vi "WinCI Query File Status.vi"(8 "error in (no error)":errorcluster, 10 "files":path[](array[path]), 11 "source control reference in":T2) -> (0 "error out":errorcluster, 1 "file status":T1[](array[typedef]), 2 "status message":string, 3 "source control reference out":T2)   [LabVIEW 2020, in "NI_SCC_WinCI.lvlib"]
uses:
  <vilib>/SourceControl/Providers/WinCI/NI_SCC_WinCI.lvlib
  <vilib>/SourceControl/sccapi/SCCAPI Refnum.ctl
  <vilib>/SourceControl/Providers/WinCI/WinCI SCC File Status.ctl
  <vilib>/SourceControl/support/SCCSup Message Strings GLBL.vi
  <vilib>/SourceControl/sccapi/NI_SCC.lvlib
panel:
  in  "null file status TD":T1
  out "raw file status":i32[](array[numeric])
  out "result":i32
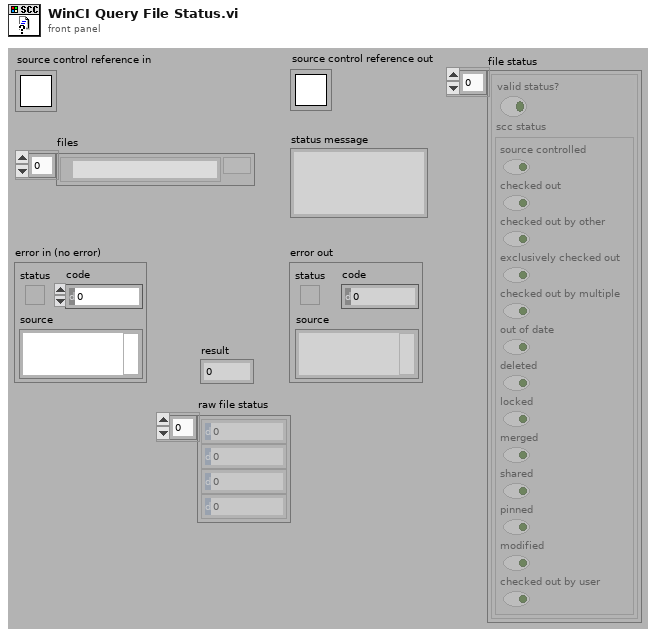
[diagram p1: front panel]
types:
  T1 = typedef "NI_SCC_WinCI.lvlib/WinCI SCC File Status.ctl" = cluster{"valid status?":bool, "scc status":cluster{"source controlled":bool, "checked out":bool, "checked out by other":bool, "exclusively checked out":bool, "checked out by multiple":bool, "out of date":bool, "deleted":bool, "locked":bool, "merged":bool, "shared":bool, "pinned":bool, "modified":bool, "checked out by user":bool}}
  T2 = typedef "NI_SCC.lvlib/SCCAPI Refnum.ctl" = refnum<k1>
  T3 = cluster{"Boolean array[0]":bool, "Boolean array[1]":bool, "Boolean array[2]":bool, "Boolean array[3]":bool, "Boolean array[4]":bool, "Boolean array[5]":bool, "Boolean array[6]":bool, "Boolean array[7]":bool, "Boolean array[8]":bool, "Boolean array[9]":bool, "Boolean array[10]":bool, "Boolean array[11]":bool, "Boolean array[12]":bool}
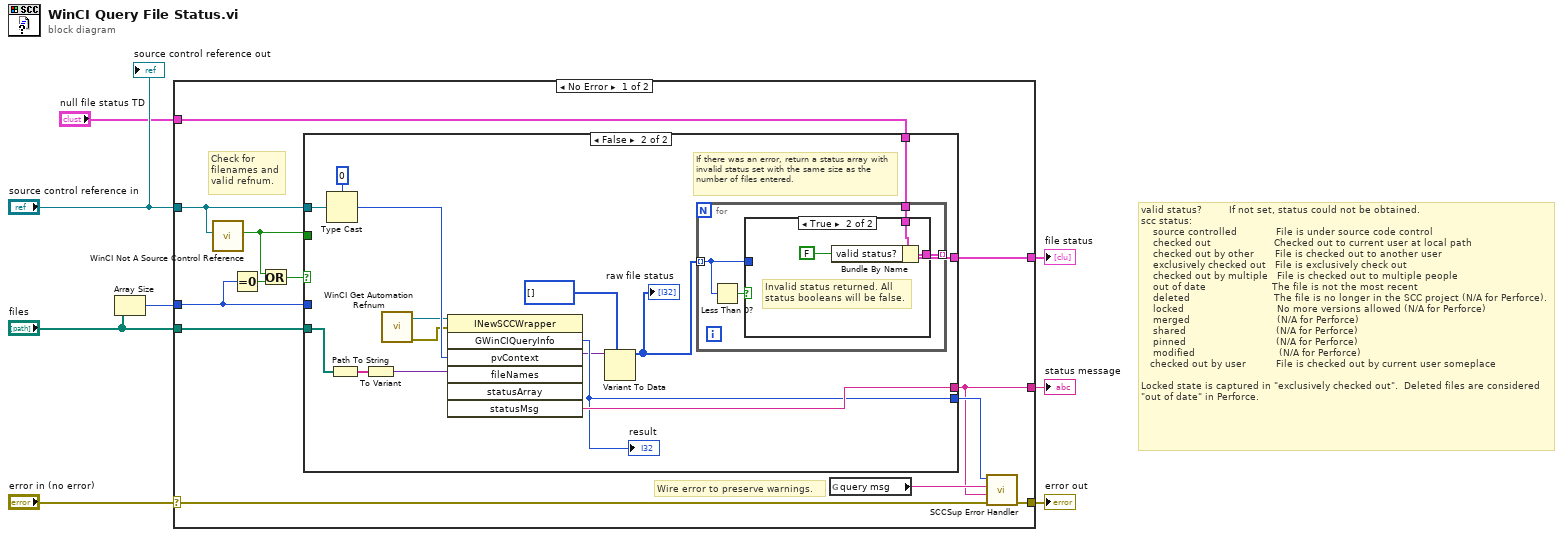
[diagram p0: block diagram]
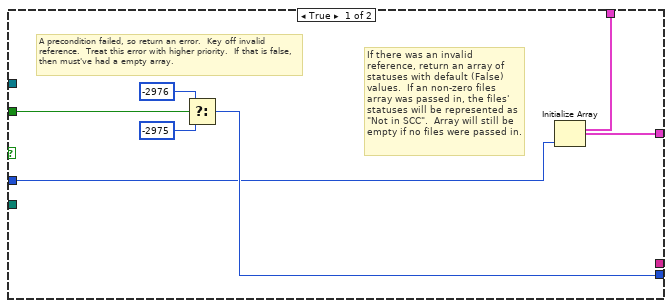
[diagram p2: hidden frame]
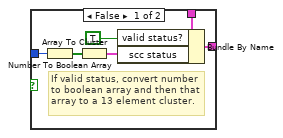
[diagram p3: hidden frame]
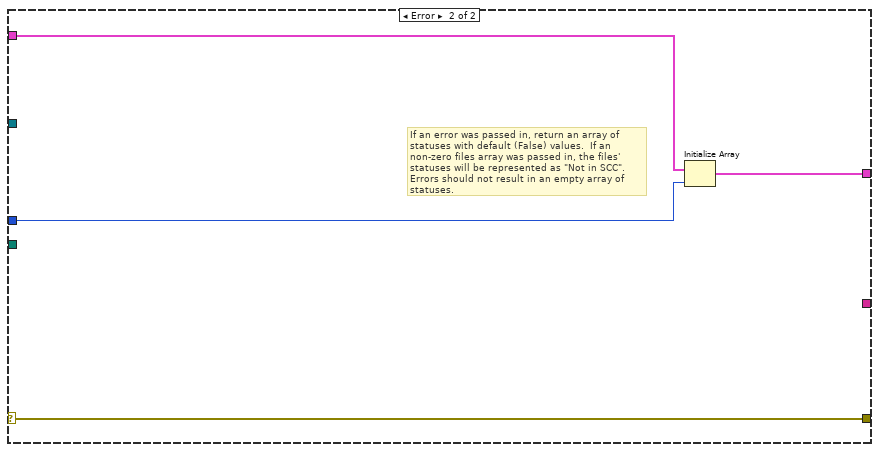
[diagram p4: hidden frame]
diagram:
  # "valid status?         If not set, status could not be obtained.\nscc status:\n    source controlled             File is under source code control\n    checked out                     Checked out to current user at local path\n    checked out by other       File is checked out to another user\n    exclusively checked out   File is exclusively check out\n    checked out by multiple   File is checked out to multiple people\n    out of date                      The file is not the most recent\n    deleted                            The file is no longer in the SCC project (N/A for Perforce). \n    locked                               No more versions allowed (N/A for Perforce)\n    merged                             (N/A for Perforce)\n    shared                              (N/A for Perforce)\n    pinned                              (N/A for Perforce)\n    modified                            (N/A for Perforce)\n   checked out by user          File is checked out by current user someplace\n\nLocked state is captured in \"exclusively checked out\".  Deleted files are considered \"out of date\" in Perforce."
  n1 = Array Size(array="files") -> (size(s)=w2:i32)
  n2 = case shown="No Error" "error in (no error)" {
    selector: "error in (no error)" -> [w13 w60]
    tunnel: [w20 w60] -> w7
    tunnel: "source control reference in" -> [w9 _]
    tunnel: [w17 _] -> w5
    tunnel: "files" -> [w15 _]
    tunnel: [w21 w59] -> w4
    tunnel: w2 -> [w12 w57]
    tunnel: "null file status TD" -> [w11 w58]
    frame No Error {
      # "Wire error to preserve warnings."
      # "Check for filenames and valid refnum."
      n3 = call <vilib>:"WinCI Not A Source Control Reference.vi"("source control reference in"=w9) -> ("not a source control reference?"=w10:bool)  [unwired: 1 in, 9 out]
      n4 = Equal To 0?(x=w12) -> (x = 0?=w16:bool)
      n5 = Or(x=w10, y=w16) -> (x .or. y?=w14:bool)
      n6 = case shown="False" w14 {
        tunnel: w9 -> [_ w43]
        tunnel: [_ w38] -> w17
        tunnel: w15 -> [_ w41]
        tunnel: [w23 w40] -> w21
        tunnel: [w25 w37] -> w19
        tunnel: w10 -> [w26 _]
        tunnel: w12 -> [w22 _]
        tunnel: w11 -> [w24 w39]
        frame True {
          # "If there was an invalid reference, return an array of statuses with default (False) values.  If an non-zero files array was passed in, the files' statuses will be represented as \"Not in SCC\".  Array will still be empty if no files were passed in."
          # "A precondition failed, so return an error.  Key off invalid reference.  Treat this error with higher priority.  If that is false, then must've had a empty array."
          n7 = Select(t=-2976 ("result"), s=w26, f=-2975 ("result")) -> (s? t:f=w25:i32)
          n8 = Initialize Array(w24, w22) -> (w23:T1[])
        }
        frame False {
          # "If there was an error, return a status array with invalid status set with the same size as the number of files entered."
          n9 = Type Cast(type=u32 0, x=w43) -> (*(type *) &x=w36:u32)
          n10 = Path To String(path=w41) -> (string=w35:string[])
          n11 = To Variant(anything=w35) -> (Variant=w34:variant)
          n12 = call <vilib>:"WinCI Get Automation Refnum.vi"() -> ("error out"=w29:errorcluster, "automation refnum"=w30:refnum<k7>)  [unwired: 10 out]
          n13 = invoke class="INewSCCWrapper" method="GWinCIQueryInfo"(reference=w30, error in=w29, "pvContext"=w36, "fileNames"=w34) -> ("GWinCIQueryInfo"=w37:i32, "statusArray"=w33:variant, "statusMsg"=w38:string)  [unwired: 3 in, 4 out]
          "result" <- w37
          n14 = Variant To Data(type=i32[] [] ("initialized array"), Variant=w33) -> (data=w31:i32[])  [unwired: 1 in, 1 out]
          "raw file status" <- w31
          n15 = for {
            tunnel: w31 -> [w44] mode=indexing
            tunnel: w39 -> [w46]
            tunnel: [w45] -> w40 mode=indexing
            n16 = Less Than 0?(x=w44) -> (x < 0?=w47:bool)
            n17 = case shown="True" w47 {
              tunnel: w46 -> [w51 w56]
              tunnel: [w49 w54] -> w45
              tunnel: w44 -> [w53 _]
              frame False {
                # "If valid status, convert number to boolean array and then that array to a 13 element cluster."
                n18 = Number To Boolean Array(number=w53) -> (Boolean array=w52:bool[])
                n19 = Array To Cluster(array=w52) -> (cluster=w50:T3)
                n20 = Bundle By Name(cluster=w51, "valid status?"=TRUE, "scc status"=w50) -> (w49:T1)
              }
              frame True {
                # "Invalid status returned. All status booleans will be false."
                n21 = Bundle By Name(cluster=w56, "valid status?"=FALSE) -> (w54:T1)
              }
            }
          }
        }
      }
      n22 = global read "SCCSup Message Strings GLBL.vi" "query msg"() -> (w18:string)
      n23 = call <vilib>:"SCCSup Error Handler.vi"("error in (no error)"=w13, "additional message"=w17, "operation message"=w18, "scc error code"=w19) -> ("error out"=w20:errorcluster)  [unwired: 7 out]
    }
    frame Error {
      # "If an error was passed in, return an array of statuses with default (False) values.  If an non-zero files array was passed in, the files' statuses will be represented as \"Not in SCC\".  Errors should not result in an empty array of statuses."
      n24 = Initialize Array(w58, w57) -> (w59:T1[])
    }
  }
  "error out" <- w7
  "status message" <- w5
  "file status" <- w4
  "source control reference out" <- "source control reference in"
